vi "Init PowerSupply.vi"(8 "error in (no error)":errorcluster, 11 "PsuVisaSim-Fix in":refnum<class "PsuVisaSim-Fix.lvclass">) -> (0 "error out":errorcluster, 3 "PsuVisaSim-Fix out":refnum<class "PsuVisaSim-Fix.lvclass">)   [LabVIEW 2020, in "LAF2024Q2.lvlib" / "PsuVisaSim-Fix.lvclass"]
uses:
  PsuVisaSim-Fix.lvclass
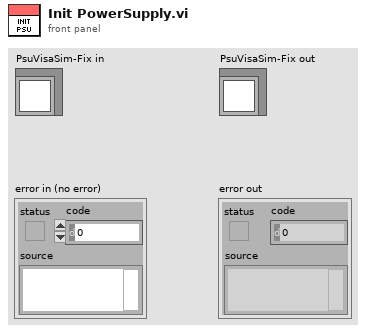
[diagram p1: front panel]
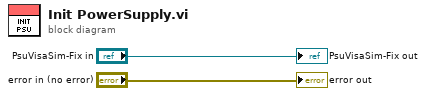
[diagram p0: block diagram]
diagram:
  "error out" <- "error in (no error)"
  "PsuVisaSim-Fix out" <- "PsuVisaSim-Fix in"
